vi "Centroid.vi"() -> ()   [LabVIEW 2017]
panel:
  out "Centroid (Target)":cluster{"X Centroid":sgl, "Y Centroid":sgl} {"Y Centroid" format="%.2f"; "X Centroid" format="%.2f"}
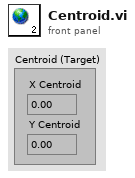
[diagram p1: front panel]
diagram:
